vi "Create Menu Bar.vi"(2 "Entry Level":T1, 5 "menubar":refnum<k9>, 11 "error in (no error)":errorcluster) -> (15 "error out":errorcluster)   [LabVIEW 2019]
doc: "Read Config.ini[Menu Bar]下的Key作為Menu Tag,Key的Value作為Menu Tag下的Tag"
uses:
  Ctrl/IDLevel.ctl
panel:
  # "Creat Menu Bar"
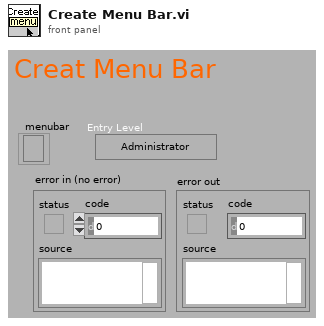
[diagram p1: front panel]
types:
  T1 = typedef "IDLevel.ctl" = enum16{"Administrator", "Engineer", "Operator", "LogIn/Out"}
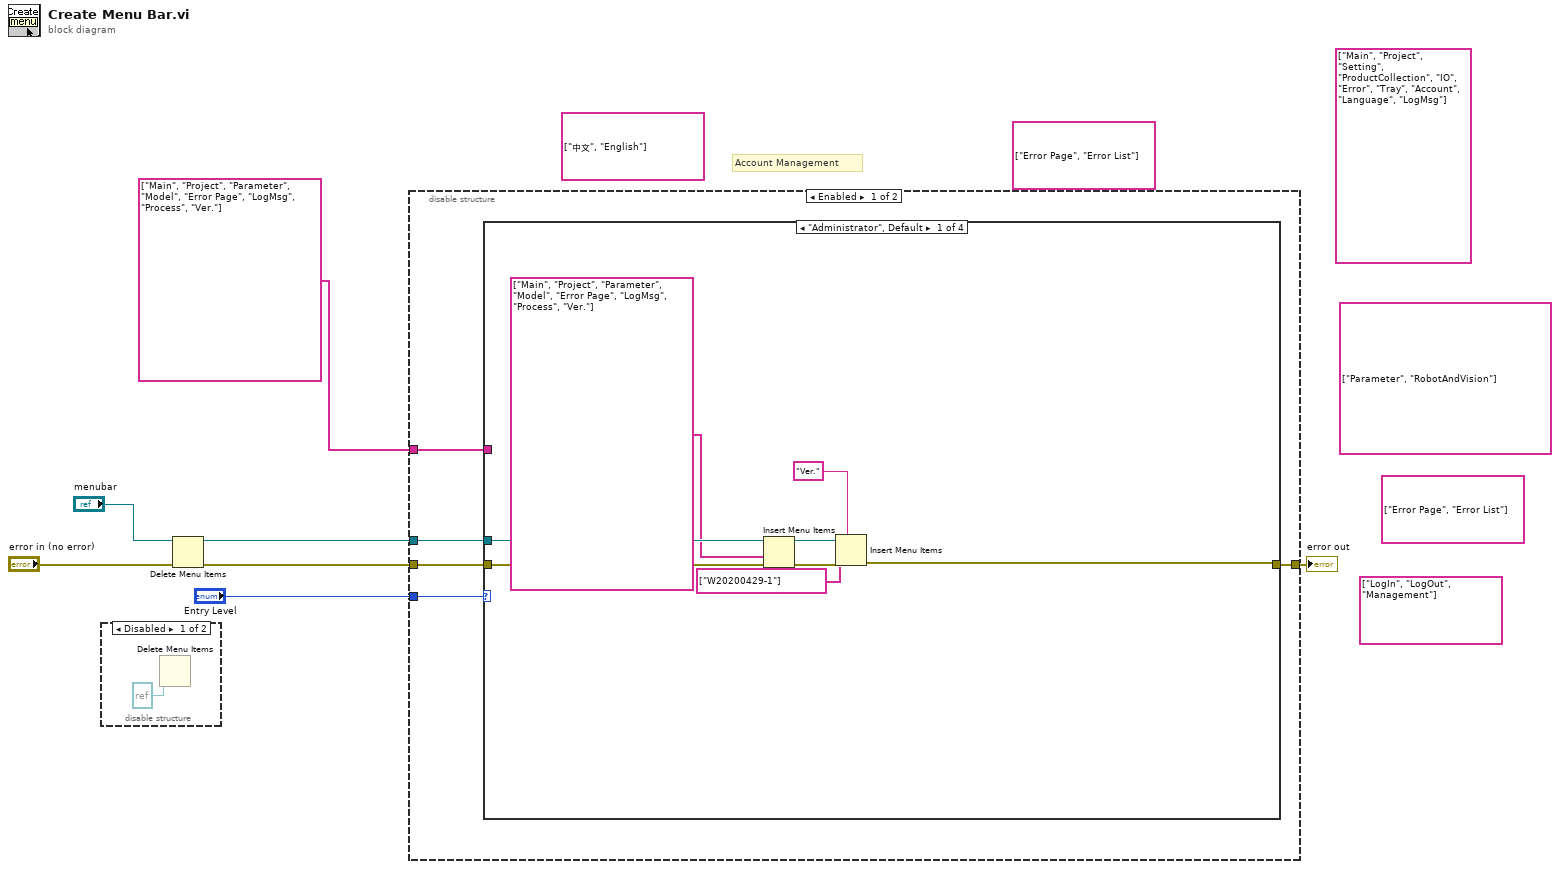
[diagram p0: block diagram]
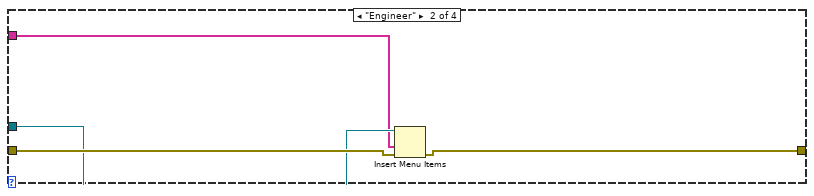
[diagram p2: hidden frame]
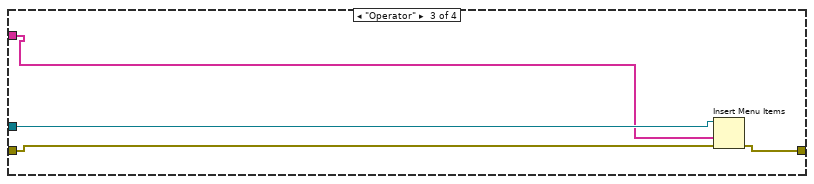
[diagram p3: hidden frame]
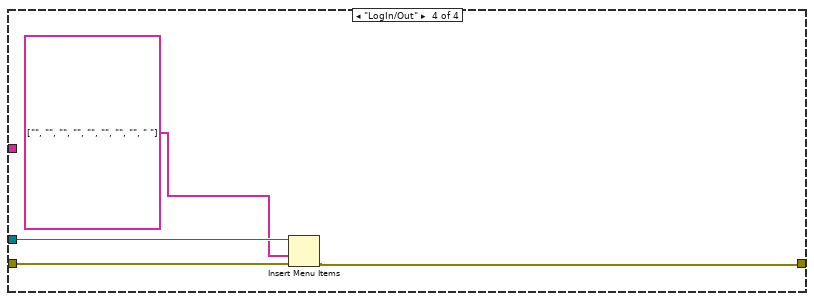
[diagram p4: hidden frame]
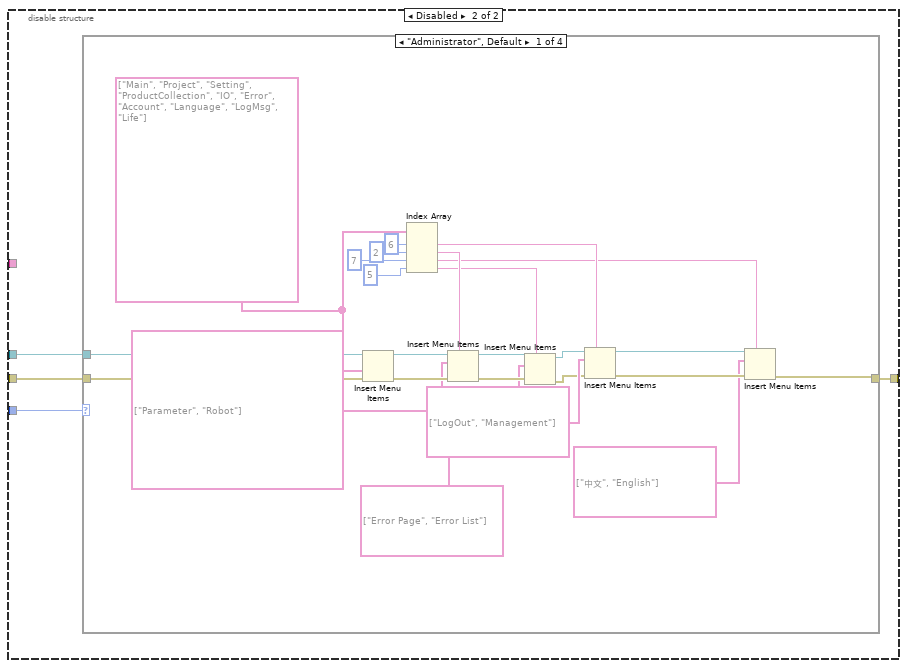
[diagram p5: hidden frame]
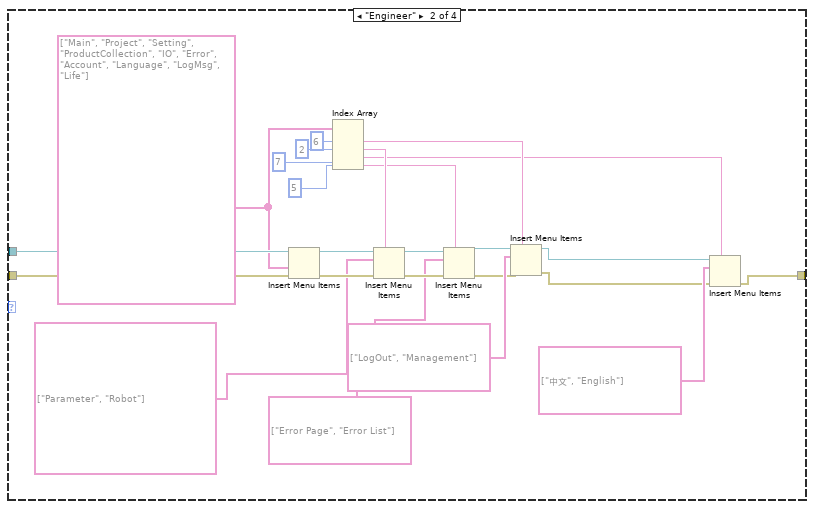
[diagram p6: hidden frame]
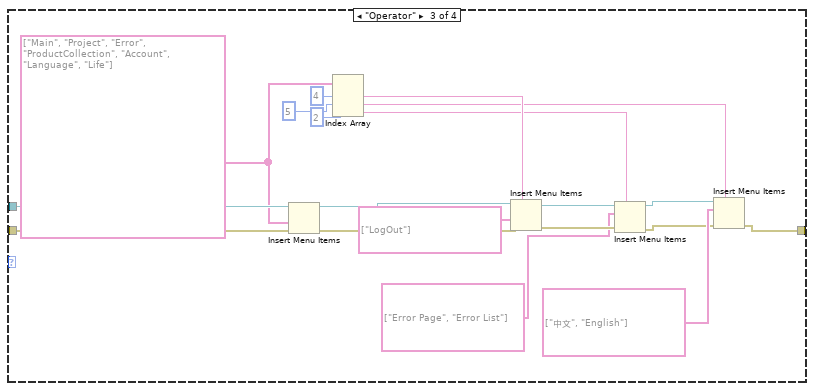
[diagram p7: hidden frame]
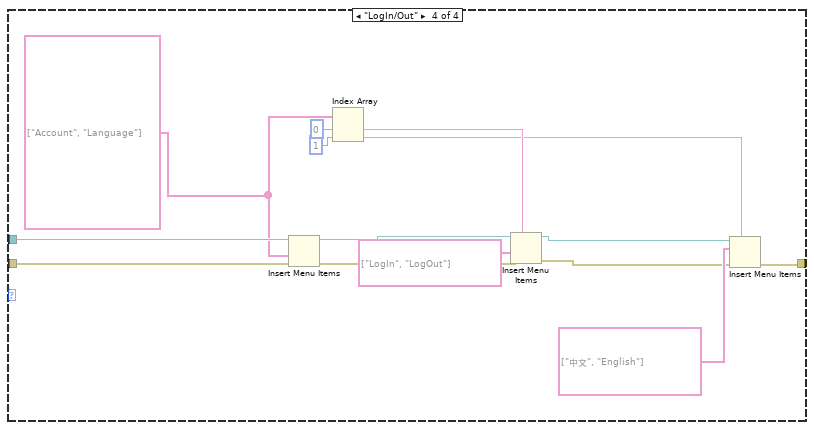
[diagram p8: hidden frame]
diagram:
  (unwired) string[] ["中文", "English"] ("item tags")
  (unwired) string[] ["LogIn", "LogOut", "Management"] ("item tags")
  (unwired) string[] ["Error Page", "Error List"] ("item tags")
  (unwired) string[] ["Parameter", "RobotAndVision"] ("item tags")
  (unwired) string[] ["Main", "Project", "Setting", "ProductCollection", "IO", "Error", "Tray", "Account", "Language", "LogMsg"] ("item tags")
  (unwired) string[] ["Error Page", "Error List"] ("item tags")
  # "Account Management"
  n1 = disable-structure shown="Disabled" {
    frame Disabled {
      n2 = Delete Menu Items(9:refnum<k9> refnum ("menu reference")) -> ()  [unwired: 2 in, 3 out]
    }
    frame Enabled {
    }
  }
  n3 = Delete Menu Items(6:"error in (no error)", 9:"menubar") -> (0:w3:errorcluster, 3:w5:refnum<k9>)  [unwired: 1 in, 1 out]
  n4 = disable-structure shown="Enabled" {
    disable-tunnel: "Entry Level" -> [w13 w37]
    disable-tunnel: w5 -> [w12 w36]
    disable-tunnel: w3 -> [w11 w35]
    disable-tunnel: [w10 w34] -> w2
    disable-tunnel: string[] ["Main", "Project", "Parameter", "Model", "Error Page", "LogMsg", "Process", "Ver."] ("item tags") -> [w9 _]
    frame Enabled {
      n5 = case shown="\"Administrator\", Default" w13 {
        tunnel: w11 -> [w20 w25 w28 w32]
        tunnel: w12 -> [w21 w23 w27 w33]
        tunnel: [w16 w24 w29 w30] -> w10
        tunnel: w9 -> [_ w22 w26 _]
        frame "Administrator", Default {
          n6 = Insert Menu Items(6:w20, 7:string[] ["Main", "Project", "Parameter", "Model", "Error Page", "LogMsg", "Process", "Ver."] ("item tags"), 9:w21) -> (0:w17:errorcluster, 3:w18:refnum<k9>)  [unwired: 4 out]
          n7 = Insert Menu Items(5:"Ver.", 6:w17, 7:string[] ["W20200429-1"] ("item tags"), 9:w18) -> (0:w16:errorcluster)  [unwired: 4 out]
        }
        frame "Engineer" {
          n8 = Insert Menu Items(6:w25, 7:w22, 9:w23) -> (0:w24:errorcluster)  [unwired: 5 out]
        }
        frame "Operator" {
          n9 = Insert Menu Items(6:w28, 7:w26, 9:w27) -> (0:w29:errorcluster)  [unwired: 3 in, 2 out]
        }
        frame "LogIn/Out" {
          n10 = Insert Menu Items(6:w32, 7:string[] ["", "", "", "", "", "", "", "", " "] ("item tags"), 9:w33) -> (0:w30:errorcluster)  [unwired: 5 out]
        }
      }
    }
    frame Disabled {
      n11 = case shown="\"Administrator\", Default" w37 {
        tunnel: w35 -> [w58 w82 w103 w117]
        tunnel: w36 -> [w59 w83 w104 w118]
        tunnel: [w49 w71 w95 w108] -> w34
        frame "Administrator", Default {
          w53 = string[] ["Main", "Project", "Setting", "ProductCollection", "IO", "Error", "Account", "Language", "LogMsg", "Life"] ("item tags")
          n12 = Insert Menu Items(6:w58, 7:w53, 9:w59) -> (0:w60:errorcluster, 3:w61:refnum<k9>)  [unwired: 4 out]
          n13 = Index Array(array=w53, index #1=6 ("index"), index #2=2 ("index"), index #3=7 ("index"), index #4=5 ("index")) -> (element #1=w52:string, element #2=w54:string, element #3=w45:string, element #4=w41:string)
          n14 = Insert Menu Items(5:w54, 6:w60, 8:string[] ["Parameter", "Robot"] ("item tags"), 9:w61) -> (0:w42:errorcluster, 3:w39:refnum<k9>)  [unwired: 3 out]
          n15 = Insert Menu Items(5:w41, 6:w42, 8:string[] ["Error Page", "Error List"] ("item tags"), 9:w39) -> (0:w43:errorcluster, 3:w38:refnum<k9>)  [unwired: 3 out]
          n16 = Insert Menu Items(5:w52, 6:w43, 8:string[] ["LogOut", "Management"] ("item tags"), 9:w38) -> (0:w48:errorcluster, 3:w50:refnum<k9>)  [unwired: 3 out]
          n17 = Insert Menu Items(5:w45, 6:w48, 8:string[] ["中文", "English"] ("item tags"), 9:w50) -> (0:w49:errorcluster)  [unwired: 1 in, 3 out]
        }
        frame "Engineer" {
          w76 = string[] ["Main", "Project", "Setting", "ProductCollection", "IO", "Error", "Account", "Language", "LogMsg", "Life"] ("item tags")
          n18 = Insert Menu Items(6:w82, 7:w76, 9:w83) -> (0:w84:errorcluster, 3:w85:refnum<k9>)  [unwired: 4 out]
          n19 = Index Array(array=w76, index #1=6 ("index"), index #2=2 ("index"), index #3=7 ("index"), index #4=5 ("index")) -> (element #1=w78:string, element #2=w79:string, element #3=w62:string, element #4=w64:string)
          n20 = Insert Menu Items(5:w79, 6:w84, 8:string[] ["Parameter", "Robot"] ("item tags"), 9:w85) -> (0:w68:errorcluster, 3:w65:refnum<k9>)  [unwired: 3 out]
          n21 = Insert Menu Items(5:w64, 6:w68, 8:string[] ["Error Page", "Error List"] ("item tags"), 9:w65) -> (0:w67:errorcluster, 3:w66:refnum<k9>)  [unwired: 3 out]
          n22 = Insert Menu Items(5:w78, 6:w67, 8:string[] ["LogOut", "Management"] ("item tags"), 9:w66) -> (0:w72:errorcluster, 3:w73:refnum<k9>)  [unwired: 3 out]
          n23 = Insert Menu Items(5:w62, 6:w72, 8:string[] ["中文", "English"] ("item tags"), 9:w73) -> (0:w71:errorcluster)  [unwired: 1 in, 3 out]
        }
        frame "Operator" {
          w102 = string[] ["Main", "Project", "Error", "ProductCollection", "Account", "Language", "Life"] ("item tags")
          n24 = Insert Menu Items(6:w103, 7:w102, 9:w104) -> (0:w98:errorcluster, 3:w99:refnum<k9>)  [unwired: 4 out]
          n25 = Index Array(array=w102, index #1=4 ("index"), index #2=5 ("index"), index #3=2 ("index")) -> (element #1=w101:string, element #2=w86:string, element #3=w92:string)
          n26 = Insert Menu Items(5:w101, 6:w98, 7:string[] ["LogOut"] ("item tags"), 9:w99) -> (0:w90:errorcluster, 3:w91:refnum<k9>)  [unwired: 1 in, 2 out]
          n27 = Insert Menu Items(5:w92, 6:w90, 8:string[] ["Error Page", "Error List"] ("item tags"), 9:w91) -> (0:w88:errorcluster, 3:w87:refnum<k9>)  [unwired: 3 out]
          n28 = Insert Menu Items(5:w86, 6:w88, 8:string[] ["中文", "English"] ("item tags"), 9:w87) -> (0:w95:errorcluster)  [unwired: 1 in, 3 out]
        }
        frame "LogIn/Out" {
          w116 = string[] ["Account", "Language"] ("item tags")
          n29 = Insert Menu Items(6:w117, 7:w116, 9:w118) -> (0:w112:errorcluster, 3:w113:refnum<k9>)  [unwired: 4 out]
          n30 = Index Array(array=w116, index #1=0 ("index"), index #2=1 ("index")) -> (element #1=w115:string, element #2=w105:string)
          n31 = Insert Menu Items(5:w115, 6:w112, 7:string[] ["LogIn", "LogOut"] ("item tags"), 9:w113) -> (0:w109:errorcluster, 3:w107:refnum<k9>)  [unwired: 1 in, 2 out]
          n32 = Insert Menu Items(5:w105, 6:w109, 8:string[] ["中文", "English"] ("item tags"), 9:w107) -> (0:w108:errorcluster)  [unwired: 1 in, 3 out]
        }
      }
    }
  }
  "error out" <- w2
